vi "3d_view.vi"(2 "3D values":T1(array[cluster]), 4 "3D Curve":refnum<k7>(container), 5 "3D view scale":dbl) -> ()   [LabVIEW 2010]
uses:
  <vilib>/Platform/NI_3dgraph.lvlib
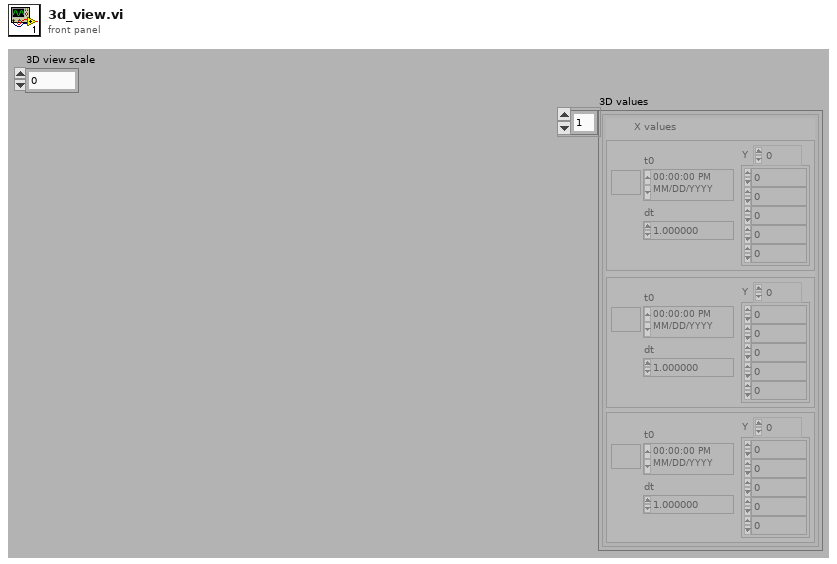
[diagram p1: front panel]
types:
  T1 = cluster{"X values":waveform(dbl), "Y values":waveform(dbl), "Z values":waveform(dbl)}[]
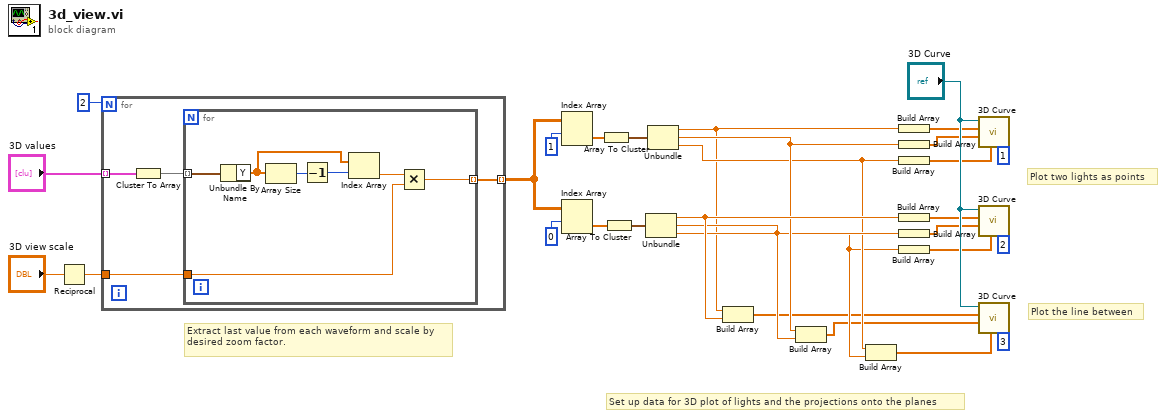
[diagram p0: block diagram]
diagram:
  # "Extract last value from each waveform and scale by desired zoom factor."
  # "Set up data for 3D plot of lights and the projections onto the planes"
  # "Plot the line between"
  # "Plot two lights as points"
  n1 = Reciprocal(x="3D view scale") -> (1/x=w6:dbl)
  n2 = for {
    N: 2 -> [_]
    tunnel: "3D values" -> [w34] mode=indexing
    tunnel: w6 -> [w32]
    tunnel: [w31] -> w5 mode=indexing
    n3 = Cluster To Array(cluster=w34) -> (array=w33:waveform(dbl)[])
    n4 = for {
      tunnel: w33 -> [w38] mode=indexing
      tunnel: w32 -> [w41]
      tunnel: [w35] -> w31 mode=indexing
      n5 = Unbundle By Name(w38) -> ("Y"=w37:dbl[])
      n6 = Array Size(array=w37) -> (size(s)=w40:i32)
      n7 = Decrement(x=w40) -> (x-1=w39:i32)
      n8 = Index Array(array=w37, index=w39) -> (element=w36:dbl)
      n9 = Multiply(x=w36, y=w41) -> (x*y=w35:dbl)
    }
  }
  n10 = Index Array(array=w5, index (row)=1 ("index")) -> (element=w4:dbl[])  [unwired: 1 in]
  n11 = Index Array(array=w5, index (row)=0 ("index")) -> (element=w1:dbl[])  [unwired: 1 in]
  n12 = Array To Cluster(array=w4) -> (cluster=w3:cluster{"[0]":dbl, "[1]":dbl, "[2]":dbl})
  n13 = Array To Cluster(array=w1) -> (cluster=w2:cluster{"[0]":dbl, "[1]":dbl, "[2]":dbl})
  n14 = Unbundle(w2) -> ("[0]"=w24:dbl, "[1]"=w20:dbl, "[2]"=w17:dbl)
  n15 = Unbundle(w3) -> ("[0]"=w10:dbl, "[1]"=w23:dbl, "[2]"=w18:dbl)
  n16 = Build Array(w10, w24) -> (w16:dbl[])
  n17 = Build Array(w23, w20) -> (w15:dbl[])
  n18 = Build Array(w18, w17) -> (w22:dbl[])
  n19 = Build Array(w10) -> (w12:dbl[])
  n20 = Build Array(w23) -> (w11:dbl[])
  n21 = Build Array(w18) -> (w21:dbl[])
  n22 = Build Array(w24) -> (w14:dbl[])
  n23 = Build Array(w20) -> (w13:dbl[])
  n24 = Build Array(w17) -> (w19:dbl[])
  n25 = call <vilib>:"3D Curve.vi"("plot number (1)"=1, "z vector"=w21, "y vector"=w11, "x vector"=w12, "3D graph"="3D Curve") -> ()  [unwired: 1 in, 6 out]
  n26 = call <vilib>:"3D Curve.vi"("plot number (1)"=2, "z vector"=w19, "y vector"=w13, "x vector"=w14, "3D graph"="3D Curve") -> ()  [unwired: 1 in, 6 out]
  n27 = call <vilib>:"3D Curve.vi"("plot number (1)"=3, "z vector"=w22, "y vector"=w15, "x vector"=w16, "3D graph"="3D Curve") -> ()  [unwired: 1 in, 6 out]
